vi "OAT Extract Most Significant Order Waveforms.vi"(0 "scaled signal [EU]":waveform(dbl)={"t0"=timestamp(0 s since 1904-01-01), "dt"=0.0, "Y"=[]}, 5 "speed profile":T3 {"speed [RPM]" format="%.2f"; "time [s]" format="%.2f"}, 9 "number of orders (3)":i32=3, 11 "error in (no error)":errorcluster, 12 "bandwidth":T2={"bandwidth value"=0.5, "bandwidth unit"=enum."Order"} {"bandwidth value" min=0.0 format="%.2f"}, 13 "window info":T1={"window type"=62, "window length"=2048} {"window type" items=["None"=0, "Hanning"=1, "Hamming"=2, "Blackman-Harris"=3, "Exact Blackman"=4, "Blackman"=5, "Flat Top"=6, "4 Term B-Harris"=7, "7 Term B-Harris"=8, "Low Sidelobe"=9, "Gaussian"=62]; "window length" min=0}) -> (4 "order waveforms [EU]":waveform(dbl)[](array[waveform]), 6 "orders":dbl[](array[numeric]) format="%.2f", 10 "unit label":string, 14 "actual window info":T1={"window type"=10, "window length"=2048} {"window type" items=["None"=0, "Hanning"=1, "Hamming"=2, "Blackman-Harris"=3, "Exact Blackman"=4, "Blackman"=5, "Flat Top"=6, "4 Term B-Harris"=7, "7 Term B-Harris"=8, "Low Sidelobe"=9, "Gaussian"=62]; "window length" min=0}, 15 "error out":errorcluster)   [LabVIEW 2017, in "SoundVib_Gabor.lvlib"]
doc: "Extracts the order waveforms with the highest power. Use this VI to examine the most influential order waveforms in a signal. This VI does not maintain state internally; you can use this VI in a loop to process multiple blocks."
uses:
  <vilib>/addons/Sound and Vibration/Order Analysis/Gabor Order Tracking/SoundVib_Gabor.lvlib
  <vilib>/addons/Sound and Vibration/Order Analysis/Tach Process/SubVIs/speed profile.ctl
  <vilib>/addons/Sound and Vibration/Order Analysis/Ref Gabor Order Tracking/Mask Bandwidth.ctl
  <vilib>/addons/Sound and Vibration/Order Analysis/Ref Gabor Order Tracking/window information.ctl
  <vilib>/addons/Sound and Vibration/Order Analysis/Ref Gabor Order Tracking/Get Order-RPM Spectral Map (DBL).vi
  <vilib>/addons/_NISVFA/_Shared subVIs/Common/svc_Engineering Units to Unit Label.vi
  <vilib>/addons/_NISVFA/_Shared subVIs/Common/svc_Unit Label to Engineering Units.vi
  <vilib>/addons/Sound and Vibration/Order Analysis/Tach Process/SoundVib_TachProcess.lvlib
panel:
  in  "Array":waveform(dbl)[](array[waveform])
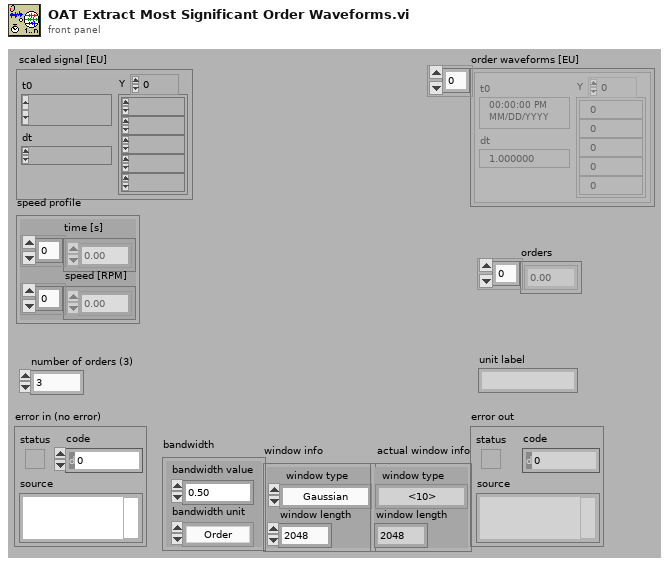
[diagram p1: front panel]
types:
  T1 = typedef "SoundVib_Gabor.lvlib/window information.ctl" = cluster{"window type":u32, "window length":i32}
  T2 = typedef "SoundVib_Gabor.lvlib/Mask Bandwidth.ctl" = cluster{"bandwidth value":dbl, "bandwidth unit":enum16{"Order", "Hz"}}
  T3 = typedef "SoundVib_TachProcess.lvlib/speed profile.ctl" = cluster{"time [s]":dbl[], "speed [RPM]":dbl[]}
  T4 = cluster{"minimum":dbl, "maximum":dbl, "increment":dbl}
  T5 = typedef "svc_Channel Info.ctl" = cluster{"sensor sensitivity":dbl, "engineering units":T6, "dB reference":dbl, "custom label":string, "weighting filter":T7, "pregain":dbl}
  T6 = typedef "svc_Engineering Units Text Ring.ctl" = u16
  T7 = typedef "svc_Weighting Filter Text Ring.ctl" = u16
  T8 = typedef "SoundVib_Gabor.lvlib/GT RefNum.ctl" = refnum<k1>
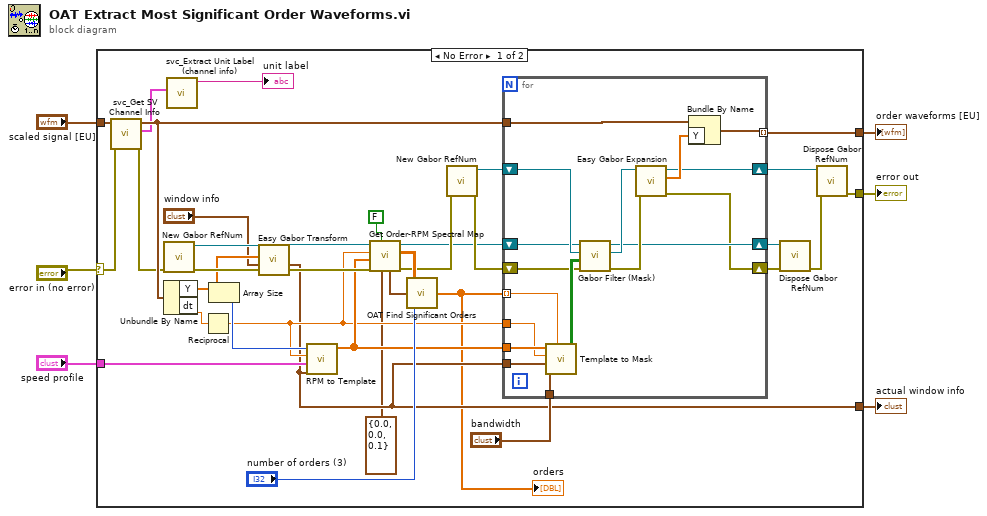
[diagram p0: block diagram]
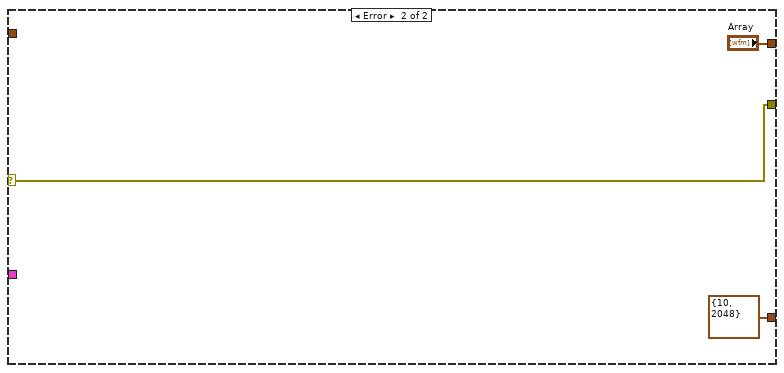
[diagram p2: hidden frame]
diagram:
  n1 = case shown="No Error" "error in (no error)" {
    selector: "error in (no error)" -> [w8 w61]
    tunnel: [w28 w61] -> w6
    tunnel: "speed profile" -> [w27 _]
    tunnel: [w24 "Array"] -> w4
    tunnel: [w18 T1 {"window type"=10, "window length"=2048} ("actual window")] -> w3
    tunnel: "scaled signal [EU]" -> [w17 _]
    frame No Error {
      n2 = call <vilib>:"svc_Get SV Channel Info.vi"("error in (no error)"=w8, "scaled signal [EU]"=w17) -> ("error out"=w7:errorcluster, "channel info"=w15:T5, "dup scaled signal [EU]"=w16:waveform(dbl))  [unwired: 4 in, 3 out]
      n3 = call <vilib>:"New Gabor RefNum.vi"("error in (no error)"=w7) -> ("error out"=w40:errorcluster, "RefNum"=w41:T8)  [unwired: 8 in]
      n4 = Unbundle By Name(w16) -> ("Y"=w23:dbl[], "dt"=w22:dbl)
      n5 = call <vilib>:"svc_Extract Unit Label (channel info).vi"("channel info"=w15) -> ("unit label"=→"unit label":string)  [unwired: 8 in, 2 out]
      n6 = Reciprocal(x=w22) -> (1/x=w21:dbl)
      n7 = Array Size(array=w23) -> (size(s)=w31:i32)
      n8 = call <vilib>:"Easy Gabor Transform.vi"("error in (no error)"=w40, "window info"="window info", "x[n]"=w23, "RefNum in"=w41) -> ("error out"=w38:errorcluster, "actual window"=w18:T1, "RefNum out"=w39:T8)  [unwired: 3 in, 2 out]
      n9 = call <vilib>:"RPM to Template.vi"("window info"=w18, "speed profile"=w27, "sampling frequency [Hz]"=w21, "signal length"=w31) -> ("Gabor template"=w26:dbl[])  [unwired: 6 in, 1 out]
      n10 = call-poly <vilib>:"Get Order-RPM Spectral Map.vi"("order range (auto)"=T4 {"minimum"=0.0, "maximum"=0.0, "increment"=0.1}, "dB On (T)"=FALSE ("log scale?"), "error in (no error)"=w38, "Gabor template"=w26, "sampling frequency [Hz]"=w21, "RefNum in"=w39) -> ("error out"=w33:errorcluster, "spectral map"=w36:dbl[][], "RefNum out"=w10:T8, "order scale"=w35:cluster{"offset":dbl, "multiplier":dbl})  [unwired: 2 out]
      n11 = call <vilib>:"OAT Find Significant Orders.vi"("num of significant orders"="number of orders (3)", "order scale"=w35, "order spectrum"=w36) -> ("orders"=w13:dbl[])
      "orders" <- w13
      n12 = call <vilib>:"New Gabor RefNum.vi"("error in (no error)"=w33) -> ("error out"=w32:errorcluster, "RefNum"=w12:T8)  [unwired: 8 in]
      n13 = for {
        tunnel: w26 -> [w58]
        shift-right: [w42] -> w29
        shift-left: w32 -> [w55]
        tunnel: w13 -> [w56] mode=indexing
        tunnel: w18 -> [w52]
        tunnel: "bandwidth" -> [w51]
        tunnel: w21 -> [w50]
        tunnel: w16 -> [w48]
        tunnel: [w47] -> w24 mode=indexing
        shift-right: [w43] -> w11
        shift-left: w12 -> [w46]
        shift-right: [w44] -> w9
        shift-left: w10 -> [w45]
        n14 = call <vilib>:"Template to Mask.vi"("order (1.0)"=w56, "bandwidth"=w51, "window info"=w52, "sampling frequency [S/s]"=w50, "Gabor template"=w58) -> ("mask array"=w57:bool[][])  [unwired: 6 in]
        n15 = call <vilib>:"Gabor Filter (Mask).vi"("error in (no error)"=w55, "mask array"=w57, "dest RefNum in"=w46, "src RefNum in"=w45) -> ("error out"=w53:errorcluster, "dest RefNum out"=w54:T8, "RefNum out"=w44:T8)  [unwired: 5 in]
        n16 = call <vilib>:"Easy Gabor Expansion.vi"("error in (no error)"=w53, "RefNum in"=w54) -> ("error out"=w42:errorcluster, "time waveform"=w49:dbl[], "RefNum out"=w43:T8)  [unwired: 7 in]
        n17 = Bundle By Name(cluster=w48, "Y"=w49) -> (w47:waveform(dbl))
      }
      n18 = call <vilib>:"Dispose Gabor RefNum.vi"("error in (no error)"=w29, "RefNum in"=w9) -> ("error out"=w30:errorcluster)  [unwired: 6 in]
      n19 = call <vilib>:"Dispose Gabor RefNum.vi"("error in (no error)"=w30, "RefNum in"=w11) -> ("error out"=w28:errorcluster)  [unwired: 6 in]
    }
    frame Error {
    }
  }
  "error out" <- w6
  "order waveforms [EU]" <- w4
  "actual window info" <- w3
